vi "LogToXMLFile.vi"(8 "Error In":errorcluster, 11 "Spaceship In":refnum<class "Spaceship.lvclass">) -> (0 "Error Out":errorcluster, 3 "Spaceship Out":refnum<class "Spaceship.lvclass">)   [LabVIEW 2021, in "Spaceship.lvclass"]
doc: "Save specific class data to file as XML."
uses:
  Spaceship.lvclass
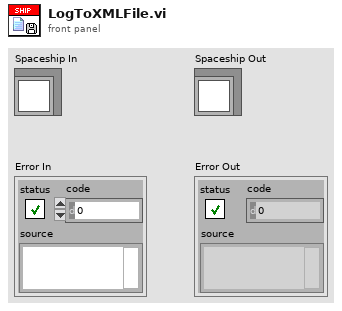
[diagram p1: front panel]
types:
  T1 = enum16{"open", "replace", "create", "open or create", "replace or create", "replace or create with confirmation"}
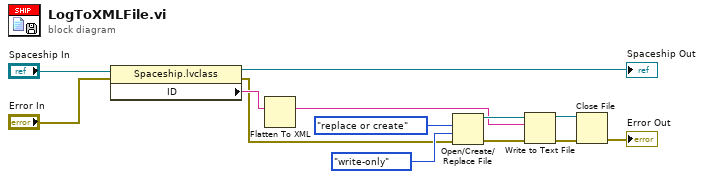
[diagram p0: block diagram]
diagram:
  n1 = property class="Spaceship.lvclass"(reference="Spaceship In", error in="Error In") -> (reference out=→"Spaceship Out":refnum<class "Spaceship.lvclass">, error out=w3:errorcluster, "ID"=w5:string)
  n2 = Flatten To XML(6:w5) -> (2:w9:string)
  n3 = Open/Create/Replace File(error in=w3, operation (0:open)=T1."replace or create", access (0:read/write)=enum16{"read/write", "read-only", "write-only"}."write-only") -> (refnum out=w10:refnum<file>, error out=w11:errorcluster)  [unwired: 3 in, 1 out]
  n4 = Write to Text File(file (use dialog)=w10, text=w9, error in=w11) -> (refnum out=w8:refnum<file>, error out=w7:errorcluster)  [unwired: 1 in, 1 out]
  n5 = Close File(refnum=w8, error in=w7) -> (error out=→"Error Out":errorcluster)  [unwired: 1 out]
